vi "Sound-Enumerate Inputs.vi"() -> (8 "Names":string[](array[string]), 15 "error out":errorcluster)   [LabVIEW 2020]
uses:
  <vilib>/Dataflow_G/G-Audio/G-Audio.lvlib
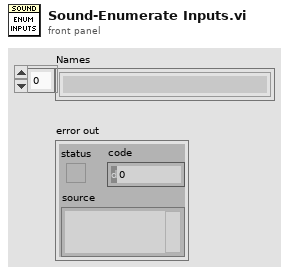
[diagram p1: front panel]
types:
  T1 = typedef "G-Audio.lvlib/Audio Device Info.ctl" = cluster{"Name":string, "ID":u8[], "Device Type":T2, "Default":bool, "Native Data Formats":T3[]}
  T2 = typedef "G-Audio.lvlib/Audio Device Type.ctl" = enum16{"(None)", "Playback", "Capture", "Duplex", "Loopback"}
  T3 = typedef "G-Audio.lvlib/Audio Device Native Data Format.ctl" = cluster{"Format":T4, "Channels":u32, "Sample Rate (Hz)":u32, "Exclusive Mode":bool}
  T4 = typedef "G-Audio.lvlib/Audio Device Format.ctl" = enum16{"Native", "U8", "I16", "I32", "SGL"}
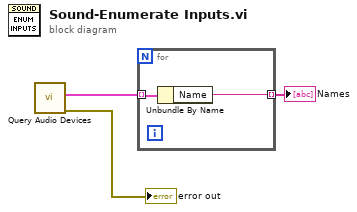
[diagram p0: block diagram]
diagram:
  n1 = call <vilib>:"Query Audio Devices.vi"() -> ("error out"=→"error out":errorcluster, "Capture Devices"=w1:T1[])  [unwired: 7 in, 3 out]
  n2 = for {
    tunnel: w1 -> [w5] mode=indexing
    tunnel: [w4] -> w2 mode=indexing
    n3 = Unbundle By Name(w5) -> ("Name"=w4:string)
  }
  "Names" <- w2
